vi "Verify Voltage Setting.vi"(8 "error in (no error)":errorcluster, 11 "N5745A in":refnum<class "N5745A.lvclass">) -> (0 "error out":errorcluster, 3 "N5745A out":refnum<class "N5745A.lvclass">)   [LabVIEW 2017, in "N5745A.lvlib" / "N5745A.lvclass"]
doc: "This method is used to verify that the N5745A Voltage setting is not greater than the manufacturer's maximum voltage rating. If greater, this method changes the voltage setting tothe manufacturer's maximum voltage rating."
uses:
  N5745A.lvclass
  N5745A.lvclass/N5745A.ctl
  PPLs/Power Supply/Parent/Power_Supply.lvlibp/Power Supply.lvclass
  C:/Projects/LabVIEW/PPLs/Power Supply/Parent/Power_Supply.lvlibp/Power Supply.lvclass
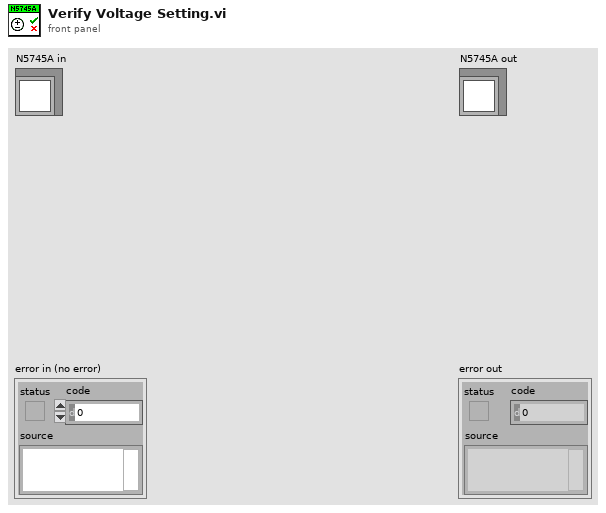
[diagram p1: front panel]
types:
  T1 = typedef "Power_Supply.lvlibp/Supply Settings.ctl" = cluster{"Voltage":dbl, "Current":dbl, "Output":bool}
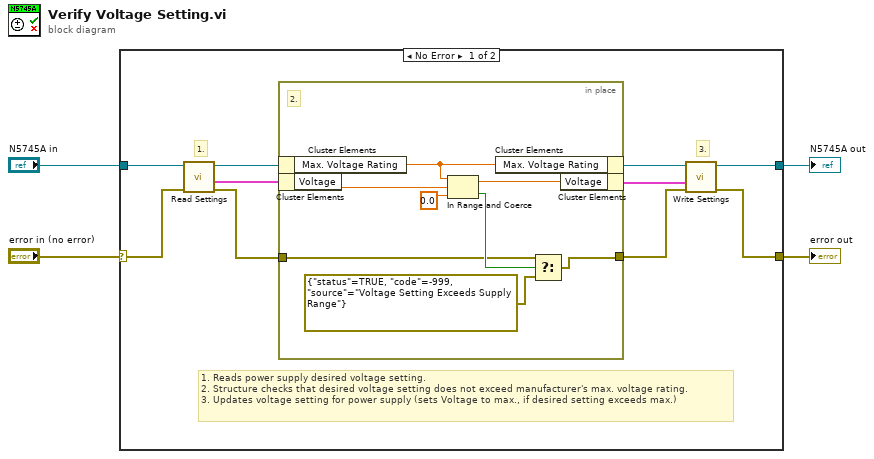
[diagram p0: block diagram]
diagram:
  n1 = case shown="No Error" "error in (no error)" {
    selector: "error in (no error)" -> [w6 w24]
    tunnel: [w10 w24] -> w3
    tunnel: [w9 w23] -> w1
    tunnel: "N5745A in" -> [w7 w23]
    frame No Error {
      # "3."
      # "1."
      # "1. Reads power supply desired voltage setting.\n2. Structure checks that desired voltage setting does not exceed manufacturer's max. voltage rating.\n3. Updates voltage setting for power supply (sets Voltage to max., if desired setting exceeds max.)"
      n2 = call "Read Settings.vi"("error in (no error)"=w6, "Power Supply in"=w7) -> ("error out"=w13:errorcluster, "Settings"=w14:T1, "Power Supply out"=w8:refnum<class "N5745A.lvclass">)  [unwired: 7 in]
      n3 = in-place {
        in-place-border: w13 -> [w19]
        in-place-border: [w17] -> w11
        # "2."
        n4 = in-place-cluster #1(w8) -> ("Max. Voltage Rating"=w15:dbl)
        n5 = in-place-cluster #2(w14) -> ("Voltage"=w22:dbl)
        n6 = In Range and Coerce(upper limit=w15, x=w22, lower limit=0.0) -> (coerced(x)=w16:dbl, In Range?=w20:bool)
        n7 = in-place-cluster #1("Max. Voltage Rating"=w15) -> (w5:refnum<class "N5745A.lvclass">)
        n8 = Select(t=w19, s=w20, f=errorcluster {"status"=TRUE, "code"=-999, "source"="Voltage Setting Exceeds Supply Range"}) -> (s? t:f=w17:errorcluster)
        n9 = in-place-cluster #2("Voltage"=w16) -> (w12:T1)
      }
      n10 = call "Write Settings.vi"("error in (no error)"=w11, "Settings"=w12, "Power Supply in"=w5) -> ("error out"=w10:errorcluster, "Power Supply out"=w9:refnum<class "N5745A.lvclass">)  [unwired: 7 in]
    }
    frame Error {
    }
  }
  "error out" <- w3
  "N5745A out" <- w1
